vi "Resolve Startup Promise.vi"(8 "error in (no error)":errorcluster, 11 "VolatusCoreTask in":refnum<class "VolatusCoreTask.lvclass">) -> (0 "error out":errorcluster, 3 "VolatusCoreTask out":refnum<class "VolatusCoreTask.lvclass">)   [LabVIEW 2020, in "Volatus.lvlib" / "VolatusCoreTask.lvclass"]
uses:
  VolatusCoreTask.lvclass
  VolatusCoreTask.lvclass/VolatusCoreTask.ctl
  lv-promises/Promises/Error Result/Error Result.lvclass
  lv-promises/Promises/Promise/Promise.lvclass
  C:/dev/lv20CE/relink/lv-promises/Promises/Value/Value.lvclass
  C:/dev/lv20CE/relink/lv-promises/Promises/Error Result/Error Result.lvclass
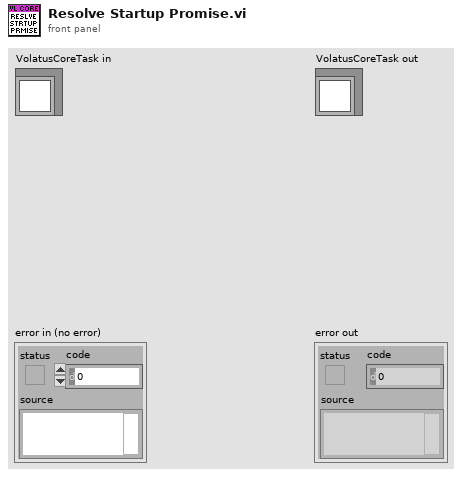
[diagram p1: front panel]
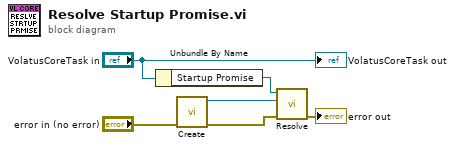
[diagram p0: block diagram]
diagram:
  n1 = Unbundle By Name("VolatusCoreTask in") -> ("Startup Promise"=w4:refnum<class "Promise.lvclass">)
  n2 = call "Create.vi"("error in (no error)"="error in (no error)") -> ("error out"=w2:errorcluster, "Error Result out"=w3:refnum<class "Error Result.lvclass">)  [unwired: 9 in]
  n3 = call "Resolve.vi"("error in (no error)"=w2, "Result"=w3, "Promise in"=w4) -> ("error out"=→"error out":errorcluster)  [unwired: 7 in, 1 out]
  "VolatusCoreTask out" <- "VolatusCoreTask in"
